vi "Write Data.vi"(6 "chip select  (1st chip)":enum16{"1st chip", "2nd chip"}(ring), 8 "error in (no error)":errorcluster, 10 "character code":u8=97 format="%.0x", 11 "LCD in":refnum<class "Character LCD.lvclass">) -> (0 "error out":errorcluster, 3 "LCD out":refnum<class "Character LCD.lvclass">)   [LabVIEW 2015, in "HD44780 Host.lvlib"]
uses:
  HD44780 Host.lvlib
  Internal/LCD Class/Character LCD.lvclass
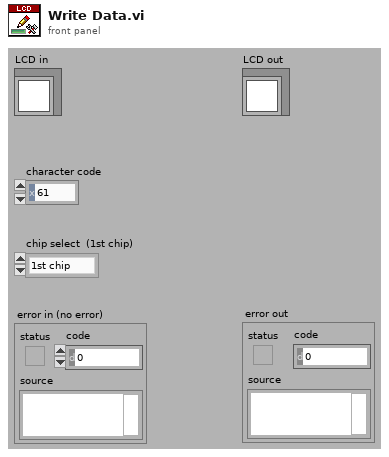
[diagram p1: front panel]
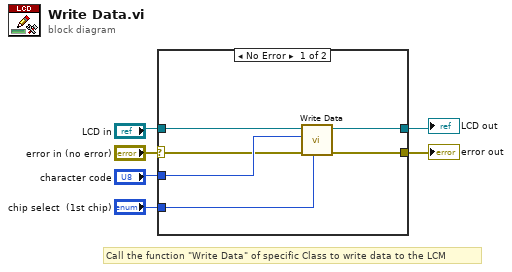
[diagram p0: block diagram]
diagram:
  # "Call the function \"Write Data\" of specific Class to write data to the LCM"
  n1 = case shown="No Error" "error in (no error)" {
    selector: "error in (no error)" -> [w7 w14]
    tunnel: "character code" -> [w12 _]
    tunnel: [w8 w14] -> w5
    tunnel: "chip select  (1st chip)" -> [w11 _]
    tunnel: "LCD in" -> [w10 w13]
    tunnel: [w9 w13] -> w1
    frame No Error {
      n2 = call-dynamic "Write Data.vi"("chip select  (1st chip)"=w11, "error in (no error)"=w7, "character code"=w12, "Character LCD in"=w10) -> ("error out"=w8:errorcluster, "Character LCD out"=w9:refnum<class "Character LCD.lvclass">)  [unwired: 6 in]
    }
    frame Error {
    }
  }
  "error out" <- w5
  "LCD out" <- w1
